vi "LVClass_WavefrontCorrector Check Actuator User Preferences.vi"(0 "WavefrontCorrector in":refnum<class "WavefrontCorrector.lvclass">, 5 "Index of actuator":i32, 7 "Wavefront Corrector State":T1, 11 "error in (no error)":errorcluster) -> (4 "WavefrontCorrector out":refnum<class "WavefrontCorrector.lvclass">, 15 "error out":errorcluster)   [LabVIEW 2020, in "WavefrontCorrector.lvclass"]
uses:
  WavefrontCorrector.lvclass
  Wavefront Corrector states - ONE.ctl
  WavefrontCorrector.lvclass/WavefrontCorrector.ctl
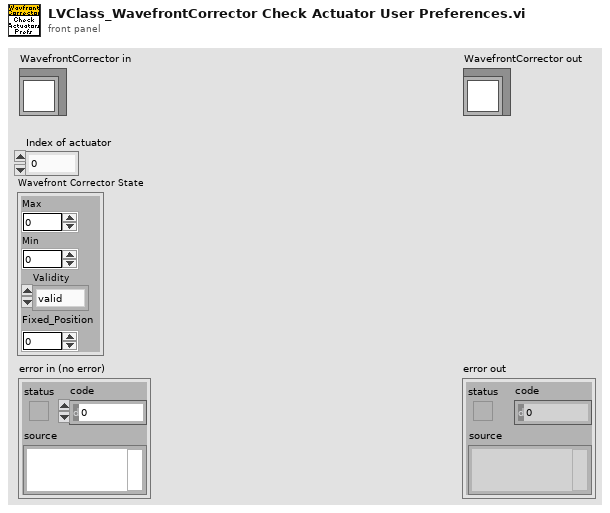
[diagram p1: front panel]
types:
  T1 = typedef "Wavefront Corrector states - ONE.ctl" = cluster{"Max":sgl, "Min":sgl, "Validity":enum16{"valid", "fixed", "invalid"}, "Fixed_Position":sgl}
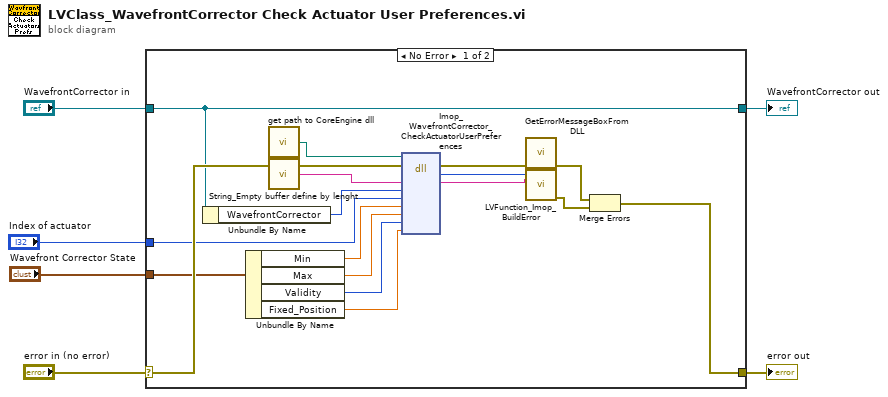
[diagram p0: block diagram]
diagram:
  n1 = case shown="No Error" "error in (no error)" {
    selector: "error in (no error)" -> [w16 w25]
    tunnel: [w15 w25] -> w5
    tunnel: [w13 w24] -> w3
    tunnel: "WavefrontCorrector in" -> [w13 w24]
    tunnel: "Wavefront Corrector State" -> [w14 _]
    tunnel: "Index of actuator" -> [w11 _]
    frame No Error {
      n2 = Unbundle By Name(w13) -> ("WavefrontCorrector"=w12:i32)
      n3 = Unbundle By Name(w14) -> ("Min"=w10:sgl, "Max"=w9:sgl, "Validity"=w8:enum16{"valid", "fixed", "invalid"}, "Fixed_Position"=w7:sgl)
      n4 = call "get path to CoreEngine dll.vi"() -> ("path to c_interface_vc100.dll"=w23:path)  [unwired: 12 in, 3 out]
      n5 = call "String_Empty buffer define by lenght.vi"() -> ("Empty buffer"=w22:string)  [unwired: 1 in]
      n6 = dll-call lib="D:/FLE/0.Code/CoreEngine4_Suite/LV2011_interface/DLLs/c_interface_vc100.dll" fn="Imop_WavefrontCorrector_CheckActuatorUserPreferences"(path in=w23, error in=w16, "Message"=w22, "WavefrontCorrector"=w12, "Index of actuator"=w11, "Min"=w10, "Max"=w9, "Validity"=w8, "Fixed position"=w7) -> (error out=w21:errorcluster, "return type"=w19:i32, "Message"=w20:string)  [unwired: 7 in, 1 out]
      n7 = call "GetErrorMessageBoxFromDLL.vi"("error IN"=w21) -> ("error OUT"=w17:errorcluster)  [unwired: 10 in]
      n8 = call "LVFunction_Imop_BuildError.vi"("code"=w19, "String to Prepend to source (\"\")"=w20) -> ("error out"=w18:errorcluster)  [unwired: 13 in]
      n9 = Merge Errors(w17, w18) -> (w15:errorcluster)
    }
    frame Error {
    }
  }
  "error out" <- w5
  "WavefrontCorrector out" <- w3
